vi "meTEC_Limit Read_ID 3000_Object Target Temperature.vi"(6 "Instance (1)":u8=1, 8 "error in (no error)":errorcluster, 9 "TEC Configuration_IN":T1={"VISA resource name"="", "Device Address"=2}, 10 "Sequence No.":u16=5552) -> (0 "error out":errorcluster, 1 "TEC Configuration_OUT":T1={"VISA resource name"="", "Device Address"=2}, 2 "Temperature Input Range_Min. [°C]":dbl, 3 "Temperature Input Range_Max. [°C]":dbl)   [LabVIEW 2019]
uses:
  TypeDefs/meTEC_Configuration.ctl
panel:
  # "--- Inputs ---"
  # "--- Outputs ---"
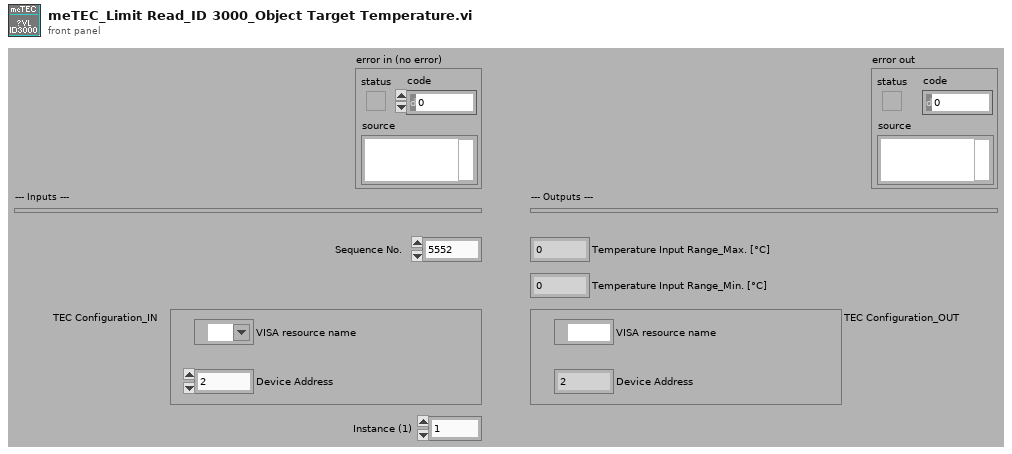
[diagram p1: front panel]
types:
  T1 = typedef "meTEC_Configuration.ctl" = cluster{"VISA resource name":refnum<visa-resource-name>, "Device Address":u16}
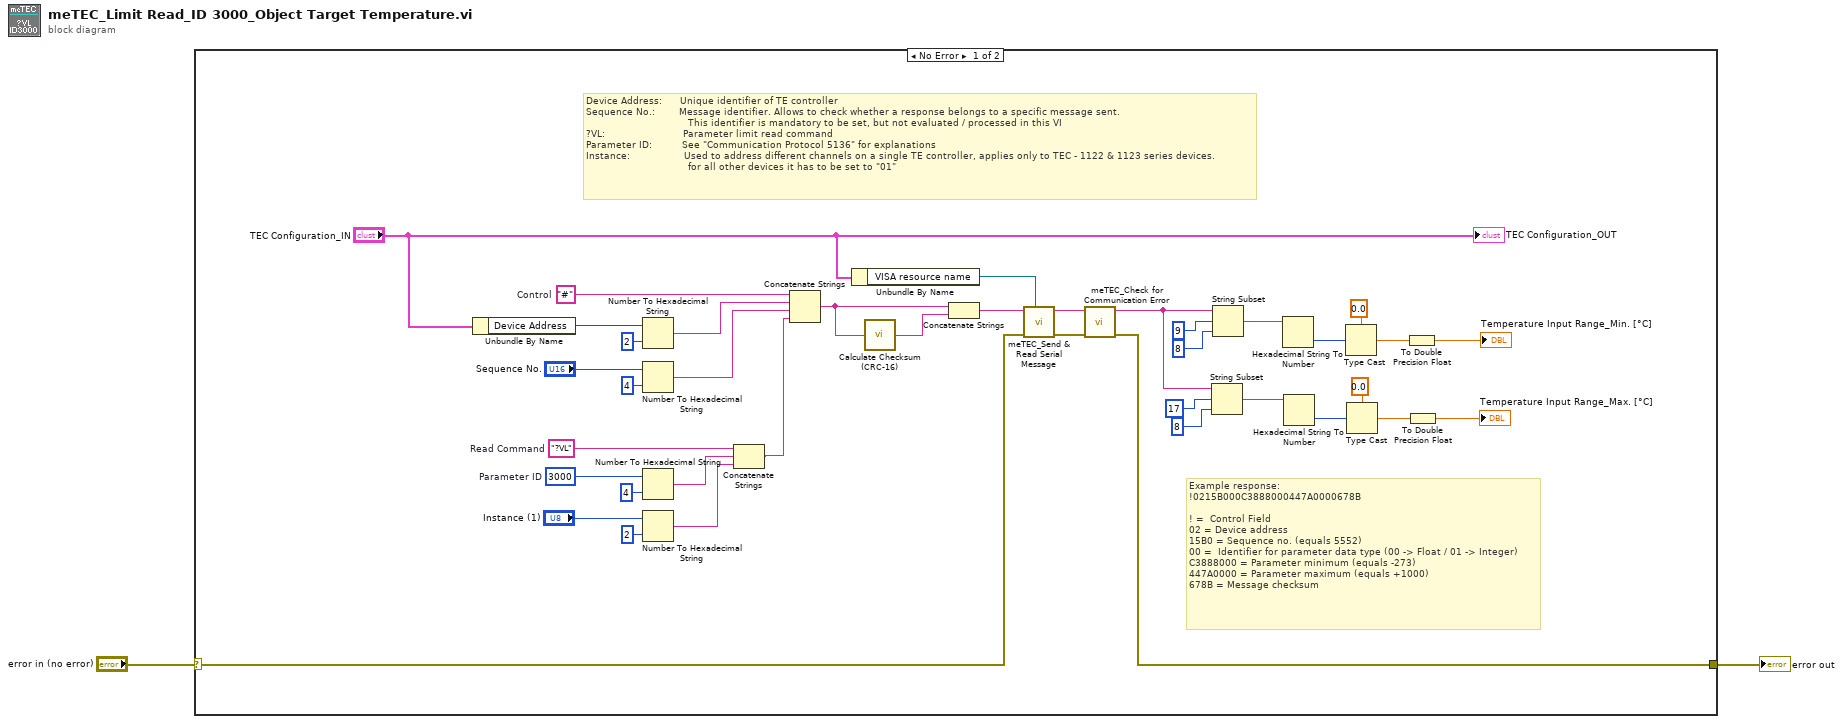
[diagram p0: block diagram]
diagram:
  n1 = case shown="No Error" "error in (no error)" {
    selector: "error in (no error)" -> [w27 w42]
    tunnel: [w19 w42] -> w2
    frame No Error {
      w30 = 3000  # Parameter ID
      w31 = "?VL"  # Read Command
      w39 = "#"  # Control
      # "Example response:\n!0215B000C3888000447A0000678B\n\n! =  Control Field\n02 = Device address\n15B0 = Sequence no. (equals 5552)\n00 =  Identifier for parameter data type (00 -> Float / 01 -> Integer)\nC3888000 = Parameter minimum (equals -273)\n447A0000 = Parameter maximum (equals +1000)\n678B = Message checksum"
      # "Device Address:      Unique identifier of TE controller\nSequence No.:        Message identifier. Allows to check whether a response belongs to a specific message sent.\n                                  This identifier is mandatory to be set, but not evaluated / processed in this VI\n?VL:                          Parameter limit read command\nParameter ID:          See \"Communication Protocol 5136\" for explanations\nInstance:                  Used to address different channels on a single TE controller, applies only to TEC - 1122 & 1123 series devices.\n                                  for all other devices it has to be set to \"01\""
      n2 = Unbundle By Name("TEC Configuration_IN") -> ("Device Address"=w22:u16)
      n3 = Number To Hexadecimal String(1:i16 2 ("width (-)"), 2:w22) -> (0:w34:string)
      n4 = Number To Hexadecimal String(1:i16 4 ("width (-)"), 2:"Sequence No.") -> (0:w38:string)
      n5 = Number To Hexadecimal String(1:i16 4 ("width (-)"), 2:w30) -> (0:w32:string)
      n6 = Number To Hexadecimal String(1:i16 2 ("width (-)"), 2:"Instance (1)") -> (0:w24:string)
      n7 = Concatenate Strings(w31, w32, w24) -> (w28:string)
      n8 = Concatenate Strings(w39, w34, w38, w28) -> (w37:string)
      n9 = Unbundle By Name("TEC Configuration_IN") -> ("VISA resource name"=w23:refnum<visa-resource-name>)
      n10 = call "Calculate Checksum (CRC-16).vi"("Message"=w37) -> ("CRC [String]"=w36:string)  [unwired: 1 in]
      n11 = Concatenate Strings(w37, w36) -> (w33:string)
      n12 = call "meTEC_Send & Read Serial Message.vi"("VISA resource name"=w23, "error in (no error)"=w27, "Serial Message"=w33) -> ("error out"=w26:errorcluster, "Serial Message_Read"=w18:string)  [unwired: 7 in]
      n13 = call "meTEC_Check for Communication Error.vi"("error in (no error)"=w26, "Serial Message_IN"=w18) -> ("error out"=w19:errorcluster, "Serial Message_OUT"=w13:string)  [unwired: 8 in]
      n14 = String Subset(string=w13, offset (0)=17, length (rest)=8 ("length (rest)")) -> (substring=w3:string)
      n15 = String Subset(string=w13, offset (0)=9, length (rest)=8 ("length (rest)")) -> (substring=w9:string)
      n16 = Hexadecimal String To Number(string=w9) -> (number=w11:u32)  [unwired: 2 in, 1 out]
      n17 = Hexadecimal String To Number(string=w3) -> (number=w7:u32)  [unwired: 2 in, 1 out]
      n18 = Type Cast(type=sgl 0.0, x=w11) -> (*(type *) &x=w12:sgl)
      n19 = Type Cast(type=sgl 0.0, x=w7) -> (*(type *) &x=w6:sgl)
      n20 = To Double Precision Float(number=w12) -> (double precision float=→"Temperature Input Range_Min. [°C]":dbl)
      n21 = To Double Precision Float(number=w6) -> (double precision float=→"Temperature Input Range_Max. [°C]":dbl)
      "TEC Configuration_OUT" <- "TEC Configuration_IN"
    }
    frame Error {
    }
  }
  "error out" <- w2
